vi "SLSC Switch Property Node.vi"   [LabVIEW 2020, in "SLSC Switch.lvlib"]
uses:
  <vilib>/SLSC_Switch/SLSC Switch.lvlib
  <resource>/objmgr/nislscsl.rc
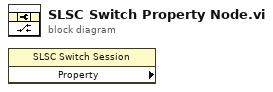
[diagram p0: block diagram]
diagram:
  n1 = property class="SLSC Switch Session" props=[]() -> ()  [unwired: 2 in, 3 out]
